vi "Get Python Location.vi"() -> (3 "path":path)   [LabVIEW 2018]
panel:
  out "error out":errorcluster
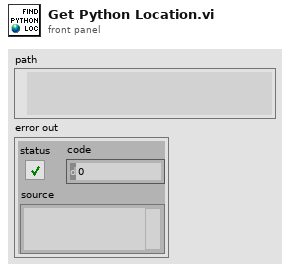
[diagram p1: front panel]
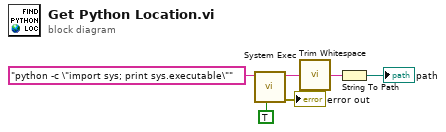
[diagram p0: block diagram]
diagram:
  n1 = call <vilib>:"System Exec.vi"("run minimized? (F)"=TRUE, "command line"="python -c \"import sys; print sys.executable\"") -> ("error out"=→"error out":errorcluster, "standard output"=w3:string)  [unwired: 6 in, 2 out]
  n2 = call <vilib>:"Trim Whitespace.vi"("string"=w3) -> ("trimmed string"=w2:string)  [unwired: 1 in]
  n3 = String To Path(string=w2) -> (path=→"path":path)
